vi "Ramp.vi"(8 "error in (no error)":errorcluster, 11 "State in":T1={"State"=enum."Idle", "Start Time"=timestamp(0 s since 1904-01-01), "Configuration"={"Cycle Period"=0.0, "Ismatech"={"VISA resource name"="", "Simulated?"=FALSE, "Pump Number"=1.0, "Reverse?"=FALSE}, "Masterflex"={"VISA resource name"="", "Simulated?"=FALSE, "Pump Number"=1.0, "Reverse?"=FALSE}, "Mettler"={"VISA resource name"="", "Simulated?"=FALSE}, "Bronkhorst M13 Flow Meter"={"VISA resource name"="", "Simulated?"=FALSE, "Smoothing Steps"=1}, "PID 2 Parameters"={"Input Device"=enum."Bronkhorst M13", "Output Device"=enum."Ismatec ISM 831C", "Setpoint"=0.0, "PID gains"={"proportional gain (Kc)"=1.0, "integral time (Ti, min)"=0.01, "derivative time (Td, min)"=0.0}}, "Manual Entry"=0.0, "Auto?"=TRUE, "PID range"={"PID High"=100.0, "PID Low"=0.0, "High Warning"=100.0}, "Tacmina Settings"={"Analog DAQ Task"="", "Digital DAQ Task"=""}, "KNF SIMDOS Settings"={"VISA resource name"="", "Simulated?"=TRUE}, "ASIA Pump C"={"ASIA Pump #"=0, "channel"=0, "Simulated"=FALSE}, "VICI Settings"={"VISA resource name"="", "Pump ID"="", "Pump Head Vol"=0.0, "Reverse?"=FALSE, "Simulated?"=FALSE}, "FLOM Settings"={"VISA resource name"="", "Simulated?"=TRUE, "Pump Number"=0.0}, "SSI PR/LD Settings"={"VISA resource name"="", "Simulated?"=FALSE}, "Masterflex 75211 Settings"={"Analog DAQ Task"="", "Digital DAQ Task"=""}, "SSI P40 Settings"={"VISA resource name"="", "Simulated?"=TRUE}, "Ismatech 3 Channel Settings"={"VISA resource name"="", "Pump Number"=1, "Channel Number"=0, "Simulated?"=TRUE, "Reverse?"=FALSE}, "Bronkhorst M14 Settings"={"VISA resource name"="", "Simulated?"=FALSE, "Smoothing Steps"=1}, "Reset Totalizer"=FALSE, "Input Num Alarm Settings"=[], "Control Type"=enum."g/min", "Front End Display Options"={"Temperature"=TRUE, "Scale Grams"=FALSE, "Density"=TRUE, "Flow (g/min)"=FALSE, "Flow (ml/min)"=TRUE, "PSIG"=TRUE, "Total Grams"=TRUE, "Updated"=TRUE}}, "Current Time"=timestamp(0 s since 1904-01-01), "PID 1 Parameters"={"Setpoint"=0.0, "PID gains"={"proportional gain (Kc)"=1.0, "integral time (Ti, min)"=0.01, "derivative time (Td, min)"=0.0}}, "First Iteration"=FALSE, "Data"={"Flowmeter (g/min)"=0.0, "Flowmeter (ml/min)"=0.0, "Density"=0.0, "FL Temp"=0.0, "Scale Output (g)"=0.0, "Scale Rate of Change (g/min)"=0.0, "PID 1 Output"=0.0, "PID 2 Process Variable"=0.0, "PID 2 output"=0.0, "Pump Flow"=0.0, "Pump Pressure"=0.0, "Totalized Value"=0.0}, "Process Name"="", "Pump On?"=enum."Off", "Input Error"=FALSE, "Output Error"=FALSE, "Log Started"=FALSE, "PID Overshoot"=FALSE, "Current Setpoint"=0.0} {"PID 1 Parameters"."PID gains"."derivative time (Td, min)" format="%.3f"; "PID 1 Parameters"."PID gains"."integral time (Ti, min)" format="%.3f"; "PID 1 Parameters"."PID gains"."proportional gain (Kc)" format="%.3f"; "Configuration"."Bronkhorst M14 Settings"."Smoothing Steps" min=1 step=1; "Configuration"."Ismatech 3 Channel Settings"."Channel Number" min=0 max=3; "Configuration"."Ismatech 3 Channel Settings"."Pump Number" min=1; "Configuration"."PID range"."PID Low" min=0.0 max=100.0 format="%.2f"; "Configuration"."PID range"."PID High" format="%.2f"; "Configuration"."PID 2 Parameters"."PID gains"."derivative time (Td, min)" format="%.3f"; "Configuration"."PID 2 Parameters"."PID gains"."integral time (Ti, min)" format="%.3f"; "Configuration"."PID 2 Parameters"."PID gains"."proportional gain (Kc)" format="%.3f"; "Configuration"."Bronkhorst M13 Flow Meter"."Smoothing Steps" min=1 step=1; "Configuration"."ASIA Pump C"."channel" min=0 max=1 step=1; "Configuration"."Ismatech"."Pump Number" min=1.0 max=20.0 step=1.0; "Configuration"."Masterflex"."Pump Number" min=1.0 max=20.0 step=1.0}) -> (0 "error out":errorcluster, 3 "State Out":T1={"State"=enum."Idle", "Start Time"=timestamp(0 s since 1904-01-01), "Configuration"={"Cycle Period"=0.0, "Ismatech"={"VISA resource name"="", "Simulated?"=FALSE, "Pump Number"=1.0, "Reverse?"=FALSE}, "Masterflex"={"VISA resource name"="", "Simulated?"=FALSE, "Pump Number"=1.0, "Reverse?"=FALSE}, "Mettler"={"VISA resource name"="", "Simulated?"=FALSE}, "Bronkhorst M13 Flow Meter"={"VISA resource name"="", "Simulated?"=FALSE, "Smoothing Steps"=1}, "PID 2 Parameters"={"Input Device"=enum."Bronkhorst M13", "Output Device"=enum."Ismatec ISM 831C", "Setpoint"=0.0, "PID gains"={"proportional gain (Kc)"=1.0, "integral time (Ti, min)"=0.01, "derivative time (Td, min)"=0.0}}, "Manual Entry"=0.0, "Auto?"=TRUE, "PID range"={"PID High"=100.0, "PID Low"=0.0, "High Warning"=100.0}, "Tacmina Settings"={"Analog DAQ Task"="", "Digital DAQ Task"=""}, "KNF SIMDOS Settings"={"VISA resource name"="", "Simulated?"=TRUE}, "ASIA Pump C"={"ASIA Pump #"=0, "channel"=0, "Simulated"=FALSE}, "VICI Settings"={"VISA resource name"="", "Pump ID"="", "Pump Head Vol"=0.0, "Reverse?"=FALSE, "Simulated?"=FALSE}, "FLOM Settings"={"VISA resource name"="", "Simulated?"=TRUE, "Pump Number"=0.0}, "SSI PR/LD Settings"={"VISA resource name"="", "Simulated?"=FALSE}, "Masterflex 75211 Settings"={"Analog DAQ Task"="", "Digital DAQ Task"=""}, "SSI P40 Settings"={"VISA resource name"="", "Simulated?"=TRUE}, "Ismatech 3 Channel Settings"={"VISA resource name"="", "Pump Number"=1, "Channel Number"=0, "Simulated?"=TRUE, "Reverse?"=FALSE}, "Bronkhorst M14 Settings"={"VISA resource name"="", "Simulated?"=FALSE, "Smoothing Steps"=1}, "Reset Totalizer"=FALSE, "Input Num Alarm Settings"=[], "Control Type"=enum."g/min", "Front End Display Options"={"Temperature"=TRUE, "Scale Grams"=FALSE, "Density"=TRUE, "Flow (g/min)"=FALSE, "Flow (ml/min)"=TRUE, "PSIG"=TRUE, "Total Grams"=TRUE, "Updated"=TRUE}}, "Current Time"=timestamp(0 s since 1904-01-01), "PID 1 Parameters"={"Setpoint"=0.0, "PID gains"={"proportional gain (Kc)"=1.0, "integral time (Ti, min)"=0.01, "derivative time (Td, min)"=0.0}}, "First Iteration"=FALSE, "Data"={"Flowmeter (g/min)"=0.0, "Flowmeter (ml/min)"=0.0, "Density"=0.0, "FL Temp"=0.0, "Scale Output (g)"=0.0, "Scale Rate of Change (g/min)"=0.0, "PID 1 Output"=0.0, "PID 2 Process Variable"=0.0, "PID 2 output"=0.0, "Pump Flow"=0.0, "Pump Pressure"=0.0, "Totalized Value"=0.0}, "Process Name"="", "Pump On?"=enum."Off", "Input Error"=FALSE, "Output Error"=FALSE, "Log Started"=FALSE, "PID Overshoot"=FALSE, "Current Setpoint"=0.0} {"PID 1 Parameters"."PID gains"."derivative time (Td, min)" format="%.3f"; "PID 1 Parameters"."PID gains"."integral time (Ti, min)" format="%.3f"; "PID 1 Parameters"."PID gains"."proportional gain (Kc)" format="%.3f"; "Configuration"."Bronkhorst M14 Settings"."Smoothing Steps" min=1 step=1; "Configuration"."Ismatech 3 Channel Settings"."Channel Number" min=0 max=3; "Configuration"."Ismatech 3 Channel Settings"."Pump Number" min=1; "Configuration"."PID range"."PID Low" min=0.0 max=100.0 format="%.2f"; "Configuration"."PID range"."PID High" format="%.2f"; "Configuration"."PID 2 Parameters"."PID gains"."derivative time (Td, min)" format="%.3f"; "Configuration"."PID 2 Parameters"."PID gains"."integral time (Ti, min)" format="%.3f"; "Configuration"."PID 2 Parameters"."PID gains"."proportional gain (Kc)" format="%.3f"; "Configuration"."Bronkhorst M13 Flow Meter"."Smoothing Steps" min=1 step=1; "Configuration"."ASIA Pump C"."channel" min=0 max=1 step=1; "Configuration"."Ismatech"."Pump Number" min=1.0 max=20.0 step=1.0; "Configuration"."Masterflex"."Pump Number" min=1.0 max=20.0 step=1.0})   [LabVIEW 2018, in "Feed Module.lvlib" / "Feed Module Engine.lvlib"]
uses:
  Feed Module Engine.lvlib
  State Cluster.ctl
  State Enum.ctl
  Feed Module/Controls/Feed Module Settings Cluster.ctl
  Ismatec ISM 831C/Controls/Ismatech ISM831C Settings Cluster.ctl
  Masterflex 7550-30/Controls/Settings Cluster.ctl
  Mettler Toledo/Controls/Settings Cluster.ctl
  Bronkhorst M13 Flow Meter/Settings Cluster.ctl
  PID 2 Parameters Cluster.ctl
  PID Input Enum.ctl
  PID 2 Output Enum.ctl
  Tacmina QI/Tacmina QI DAQ Setting.ctl
  KNF Pump/Settings Cluster plus SIMDOS.ctl
  ASIA Pump/Pump Settings.ctl
  VICI M50 Party Mode/Settings Cluster.ctl
  FLOM Pump/Settings Cluster.ctl
  SSI PR Class/SSI PR or LD Settings Cluster.ctl
  Masterflex 75211/Masterflex 75211 DAQ Setting.ctl
  SSI PR Class/SSI P40 Settings Cluster.ctl
  Ismatec 78001/Ismatec 4083.ctl
  Bronkhorst M14 Flow Meter/Settings Cluster.ctl
  Tag VIs/Numeric Alarm Settings Cluster.ctl
  PID 1 Parameters Cluster.ctl
  support/Support Library.lvlib
  Ismatec ISM 831C/Ismatec ISM 831C.lvlib
  Masterflex 7550-30/Masterflex 7550-30.lvlib
  Mettler Toledo/Mettler Toledo.lvlib
  Bronkhorst M13 Flow Meter/Bronkhorst M13 Flow Meter.lvlib
  Tacmina QI/Tacmina QI.lvlib
  KNF Pump/KNF SIMDOS.lvlib
  ASIA Pump.lvlib
  VICI M50 Party Mode/VICI M6 M50 Party Mode.lvlib
  Feed Module/Feed Module.lvlib
  FLOM Pump/FLOM Pump.lvlib
  SSI PR Class/SSI PR or LD Pump.lvlib
  Masterflex 75211/Masterflex 75211.lvlib
  SSI PR Class/SSI P40 Pump.lvlib
  Ismatec 78001/Ismatec 4308.lvlib
  Bronkhorst M14 Flow Meter/Bronkhorst M14 Flow Meter.lvlib
panel:
  in  "End":dbl
  in  "Start":dbl
  # "Output Instruments"
  # "Input Instruments"
  # "Output Instruments"
  # "Input Instruments"
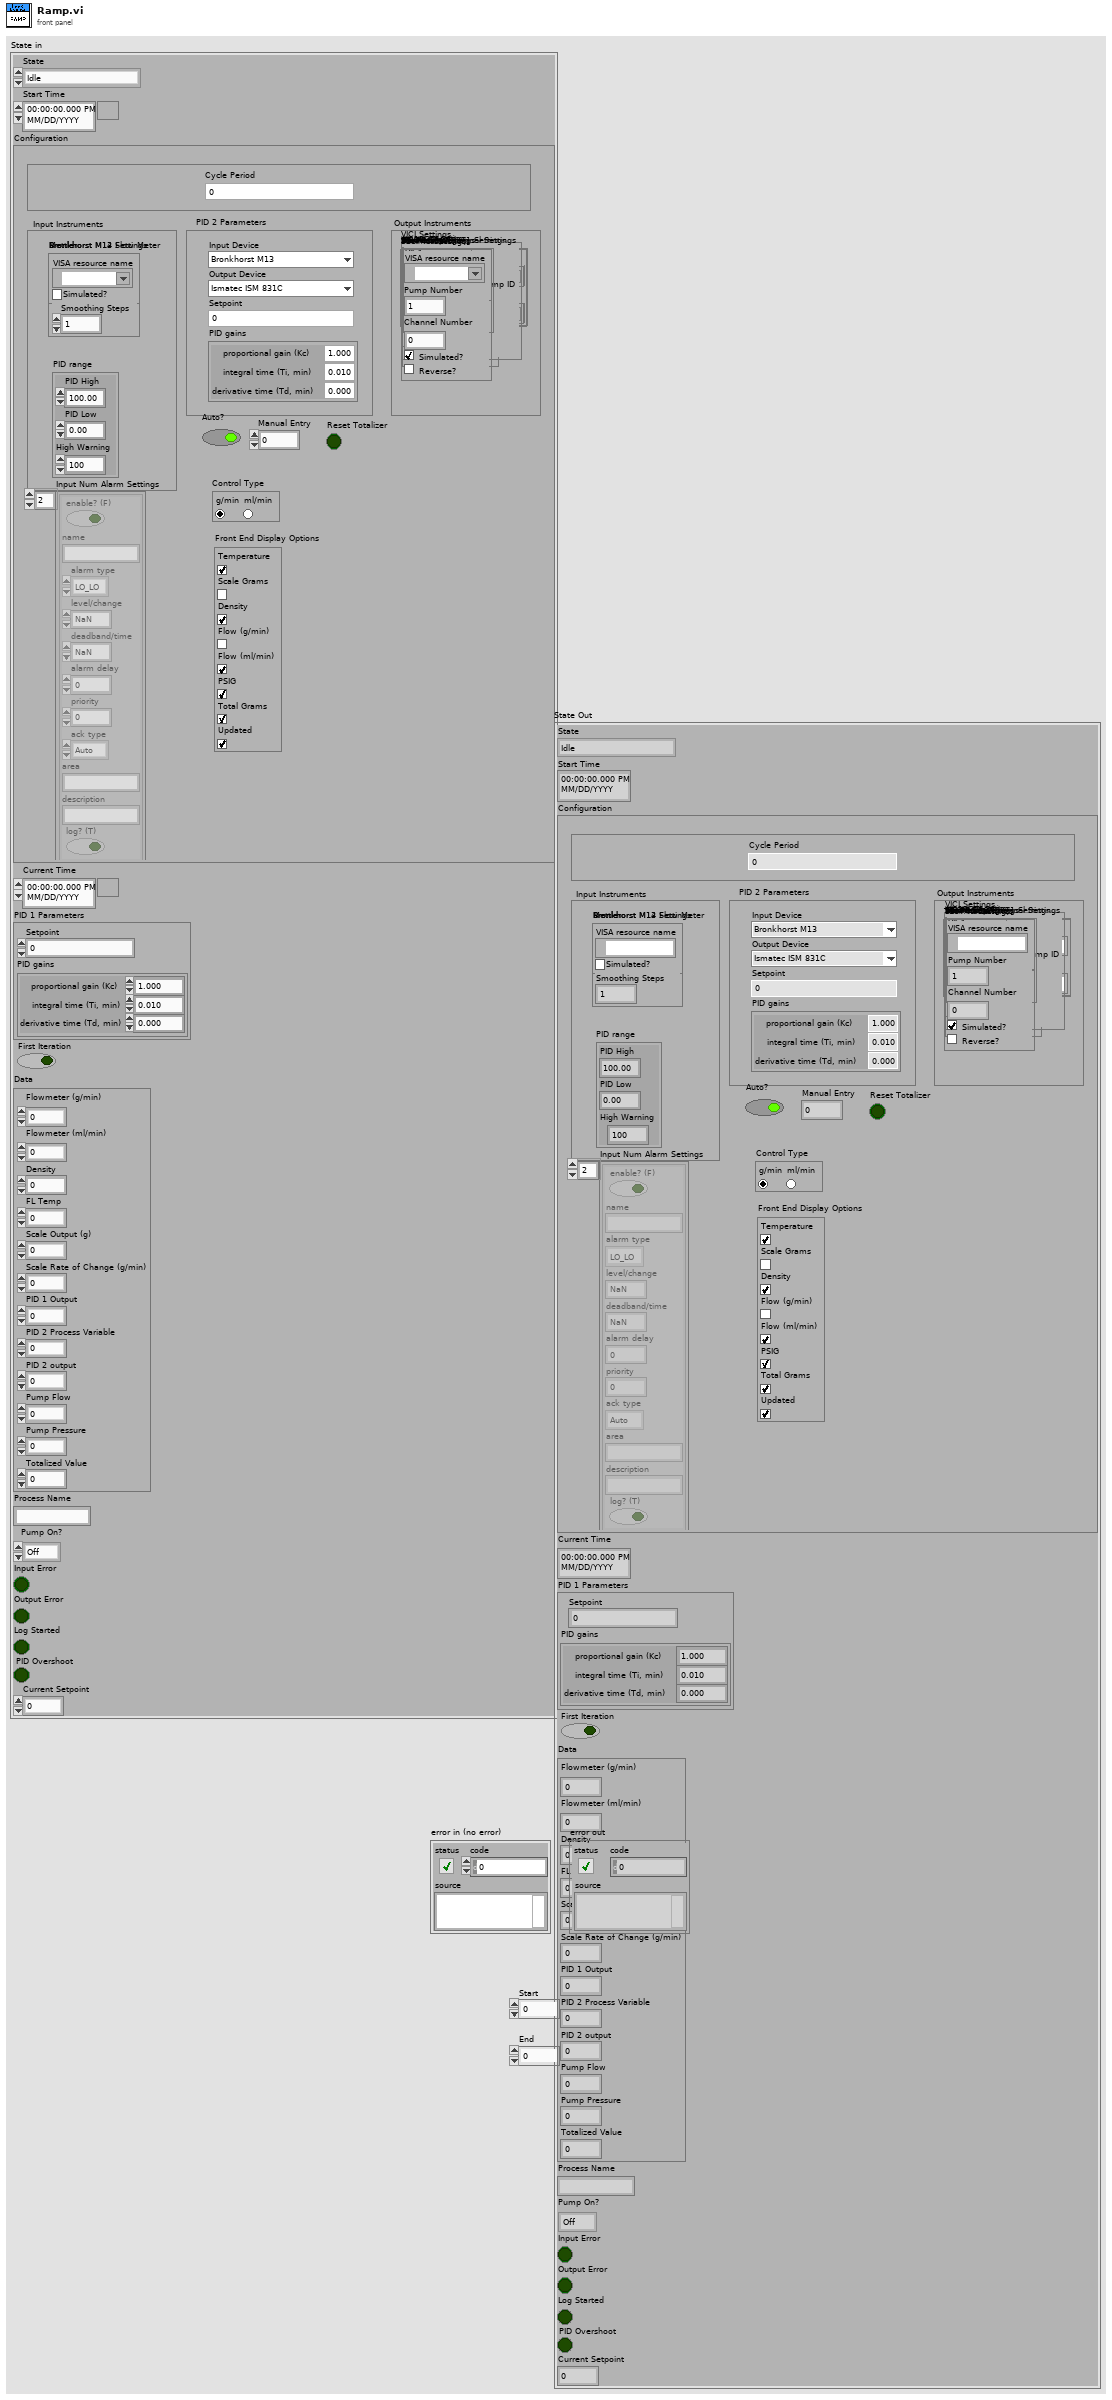
[diagram p1: front panel]
types:
  T1 = typedef "Feed Module.lvlib/Feed Module Engine.lvlib/State Cluster.ctl" = cluster{"State":T2, "Start Time":timestamp, "Configuration":T3, "Current Time":timestamp, "PID 1 Parameters":T22, "First Iteration":bool, "Data":cluster{"Flowmeter (g/min)":dbl, "Flowmeter (ml/min)":dbl, "Density":dbl, "FL Temp":dbl, "Scale Output (g)":dbl, "Scale Rate of Change (g/min)":dbl, "PID 1 Output":dbl, "PID 2 Process Variable":dbl, "PID 2 output":dbl, "Pump Flow":dbl, "Pump Pressure":dbl, "Totalized Value":dbl}, "Process Name":string, "Pump On?":enum16{"Off", "On", "Not Initialized"}, "Input Error":bool, "Output Error":bool, "Log Started":bool, "PID Overshoot":bool, "Current Setpoint":dbl}
  T2 = typedef "Feed Module.lvlib/Feed Module Engine.lvlib/State Enum.ctl" = enum16{"Measuring", "Idle", "Paused"}
  T3 = typedef "Feed Module.lvlib/Feed Module Settings Cluster.ctl" = cluster{"Cycle Period":dbl, "Ismatech":T4, "Masterflex":T5, "Mettler":T6, "Bronkhorst M13 Flow Meter":T7, "PID 2 Parameters":T8, "Manual Entry":dbl, "Auto?":bool, "PID range":cluster{"PID High":dbl, "PID Low":dbl, "High Warning":dbl}, "Tacmina Settings":T11, "KNF SIMDOS Settings":T12, "ASIA Pump C":T13, "VICI Settings":T14, "FLOM Settings":T15, "SSI PR/LD Settings":T16, "Masterflex 75211 Settings":T17, "SSI P40 Settings":T18, "Ismatech 3 Channel Settings":T19, "Bronkhorst M14 Settings":T20, "Reset Totalizer":bool, "Input Num Alarm Settings":T21[], "Control Type":enum32{"g/min", "ml/min"}, "Front End Display Options":cluster{"Temperature":bool, "Scale Grams":bool, "Density":bool, "Flow (g/min)":bool, "Flow (ml/min)":bool, "PSIG":bool, "Total Grams":bool, "Updated":bool}}
  T4 = typedef "Ismatec ISM 831C.lvlib/Ismatech ISM831C Settings Cluster.ctl" = cluster{"VISA resource name":refnum<visa-resource-name>, "Simulated?":bool, "Pump Number":dbl, "Reverse?":bool}
  T5 = typedef "Masterflex 7550-30.lvlib/Settings Cluster.ctl" = cluster{"VISA resource name":refnum<visa-resource-name>, "Simulated?":bool, "Pump Number":dbl, "Reverse?":bool}
  T6 = typedef "Mettler Toledo.lvlib/Settings Cluster.ctl" = cluster{"VISA resource name":refnum<visa-resource-name>, "Simulated?":bool}
  T7 = typedef "Bronkhorst M13 Flow Meter.lvlib/Settings Cluster.ctl" = cluster{"VISA resource name":refnum<visa-resource-name>, "Simulated?":bool, "Smoothing Steps":i32}
  T8 = typedef "PID 2 Parameters Cluster.ctl" = cluster{"Input Device":T9, "Output Device":T10, "Setpoint":dbl, "PID gains":cluster{"proportional gain (Kc)":dbl, "integral time (Ti, min)":dbl, "derivative time (Td, min)":dbl}}
  T9 = typedef "PID Input Enum.ctl" = enum16{"Default", "Bronkhorst M13", "Bronkhorst M14", "Scale Rate of Change"}
  T10 = typedef "PID 2 Output Enum.ctl" = enum16{"Default", "Ismatec ISM 4308", "Ismatec ISM 831C", "Masterflex 7550-30", "VICI M6", "VICI M50", "Tacmina QI", "KNF SIMDOS", "ASIA Type C", "FLOM UI-22-11", "SSI PR/LD", "SSI P40", "Masterflex 75211-70"}
  T11 = typedef "Tacmina QI.lvlib/Tacmina QI DAQ Setting.ctl" = cluster{"Analog DAQ Task":refnum<k21>, "Digital DAQ Task":refnum<k21>}
  T12 = typedef "KNF SIMDOS.lvlib/Settings Cluster plus SIMDOS.ctl" = cluster{"VISA resource name":refnum<visa-resource-name>, "Simulated?":bool}
  T13 = typedef "ASIA Pump.lvlib/Pump Settings.ctl" = cluster{"ASIA Pump #":i32, "channel":i32, "Simulated":bool}
  T14 = typedef "VICI M6 M50 Party Mode.lvlib/Settings Cluster.ctl" = cluster{"VISA resource name":refnum<visa-resource-name>, "Pump ID":string, "Pump Head Vol":dbl, "Reverse?":bool, "Simulated?":bool}
  T15 = typedef "FLOM Pump.lvlib/Settings Cluster.ctl" = cluster{"VISA resource name":refnum<visa-resource-name>, "Simulated?":bool, "Pump Number":dbl}
  T16 = typedef "SSI PR or LD Pump.lvlib/SSI PR or LD Settings Cluster.ctl" = cluster{"VISA resource name":refnum<visa-resource-name>, "Simulated?":bool}
  T17 = typedef "Masterflex 75211.lvlib/Masterflex 75211 DAQ Setting.ctl" = cluster{"Analog DAQ Task":refnum<k21>, "Digital DAQ Task":refnum<k21>}
  T18 = typedef "SSI P40 Pump.lvlib/SSI P40 Settings Cluster.ctl" = cluster{"VISA resource name":refnum<visa-resource-name>, "Simulated?":bool}
  T19 = typedef "Ismatec 4308.lvlib/Ismatec 4083.ctl" = cluster{"VISA resource name":refnum<visa-resource-name>, "Pump Number":i16, "Channel Number":i16, "Simulated?":bool, "Reverse?":bool}
  T20 = typedef "Bronkhorst M14 Flow Meter.lvlib/Settings Cluster.ctl" = cluster{"VISA resource name":refnum<visa-resource-name>, "Simulated?":bool, "Smoothing Steps":i32}
  T21 = typedef "Numeric Alarm Settings Cluster.ctl" = cluster{"enable? (F)":bool, "name":string, "alarm type":enum16{"HI_HI", "HI", "LO", "LO_LO"}, "level/change":dbl, "deadband/time":dbl, "alarm delay":dbl, "priority":u32, "ack type":enum16{"Auto", "User", "None", "Each Occurrence"}, "area":string, "description":string, "log? (T)":bool}
  T22 = typedef "PID 1 Parameters Cluster.ctl" = cluster{"Setpoint":dbl, "PID gains":cluster{"proportional gain (Kc)":dbl, "integral time (Ti, min)":dbl, "derivative time (Td, min)":dbl}}
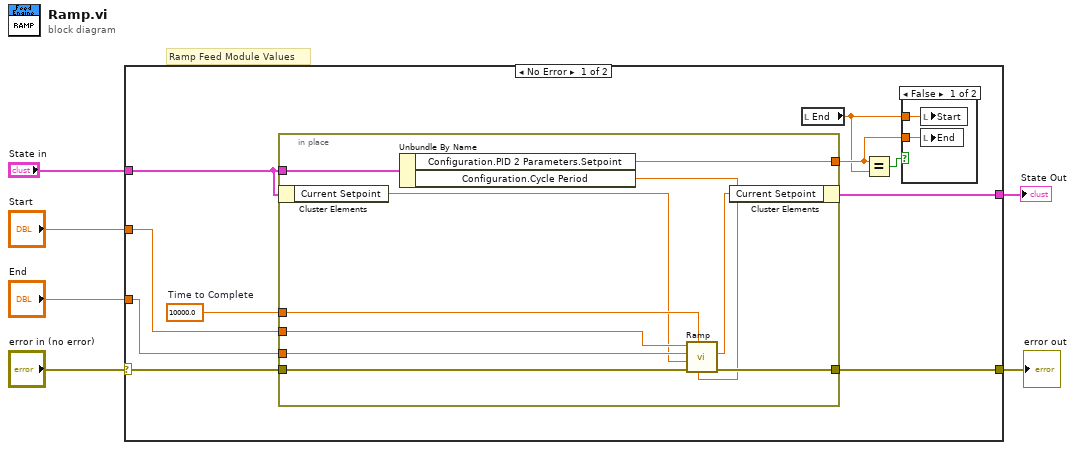
[diagram p0: block diagram]
diagram:
  # "Ramp Feed Module Values"
  n1 = case shown="No Error" "error in (no error)" {
    selector: "error in (no error)" -> [w16 w29]
    tunnel: [w15 w29] -> w5
    tunnel: "State in" -> [w8 w30]
    tunnel: [w7 w30] -> w3
    tunnel: "End" -> [w10 _]
    tunnel: "Start" -> [w9 _]
    frame No Error {
      w11 = 10000.0  # Time to Complete
      n2 = in-place {
        in-place-border: w8 -> [w26]
        in-place-border: w16 -> [w25]
        in-place-border: [w24] -> w15
        in-place-border: [w22] -> w13
        in-place-border: w11 -> [w21]
        in-place-border: w10 -> [w20]
        in-place-border: w9 -> [w19]
        n3 = in-place-cluster #1(w8) -> ("Current Setpoint"=w17:dbl)
        n4 = Unbundle By Name(w26) -> ("Configuration.PID 2 Parameters.Setpoint"=w22:dbl, "Configuration.Cycle Period"=w23:dbl)
        n5 = call "Ramp.vi"("Cycle Period"=w23, "Time to Complete"=w21, "error in (no error)"=w25, "Current"=w17, "End"=w20, "Start"=w19) -> ("error out"=w24:errorcluster, "New Current"=w18:dbl)  [unwired: 4 in]
        n6 = in-place-cluster #1("Current Setpoint"=w18) -> (w7:T1)
      }
      n7 = local read "End"() -> (w12:dbl)
      n8 = Equal?(x=w13, y=w12) -> (x = y?=w14:bool)
      n9 = case shown="False" w14 {
        tunnel: w13 -> [w28 _]
        tunnel: w12 -> [w27 _]
        frame False {
          n10 = local write "Start"(w27) -> ()
          n11 = local write "End"(w28) -> ()
        }
        frame True {
        }
      }
    }
    frame Error {
    }
  }
  "State Out" <- w3
  "error out" <- w5
